vi "DSF.Engine.Sequencer.Get Plugin Bundles.vi"(8 "error in (no error)":errorcluster, 11 "Sequencer in":refnum<class "DSF.Engine.Sequencer.lvclass">) -> (0 "error out":errorcluster, 2 "Plugin Bundles":refnum<class "DSF.Engine.Sequencer Bundle.lvclass">[](array[class]), 3 "Sequencer out":refnum<class "DSF.Engine.Sequencer.lvclass">)   [LabVIEW 2016, in "DSF.Engine.lvlib" / "DSF.Engine.Sequencer.lvclass"]
uses:
  DSF.Engine.Sequencer.lvclass
  DSF.Engine.Sequencer Bundle.lvclass
  DSF.Engine.Sequencer.lvclass/DSF.Engine.Sequencer.ctl
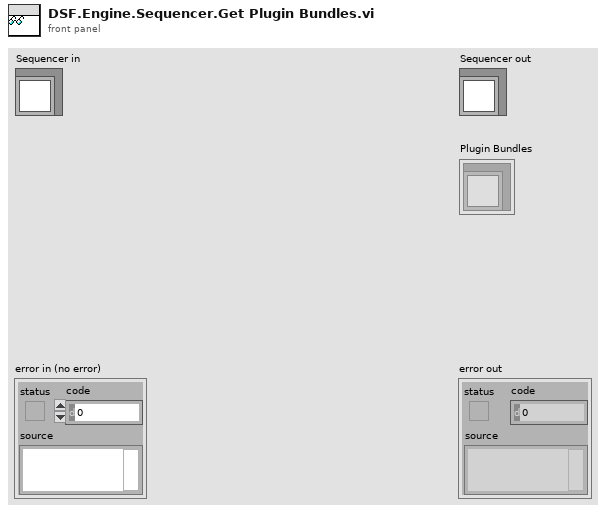
[diagram p1: front panel]
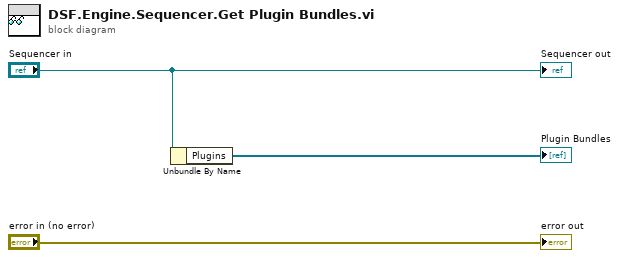
[diagram p0: block diagram]
diagram:
  n1 = Unbundle By Name("Sequencer in") -> ("Plugins"=→"Plugin Bundles":refnum<class "DSF.Engine.Sequencer Bundle.lvclass">[])
  "error out" <- "error in (no error)"
  "Sequencer out" <- "Sequencer in"
